vi "Initialize_Filtering_Settings-3.vi"(1 "Sigma #2":dbl, 2 "Sigma #1":dbl) -> (0 "[OUT] Filtering Settings":T1)   [LabVIEW 2013]
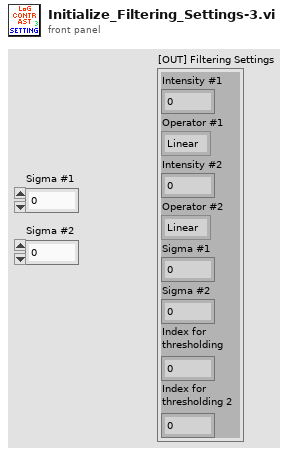
[diagram p1: front panel]
types:
  T1 = cluster{"Intensity #1":sgl, "Operator #1":enum32{"Linear", "Log", "Exp", "Square", "Square root", "Power X", "Power 1/X"}, "Intensity #2":sgl, "Operator #2":enum32{"Linear", "Log", "Exp", "Square", "Square root", "Power X", "Power 1/X"}, "Sigma #1":dbl, "Sigma #2":dbl, "Index for \nthresholding":u8, "Index for \nthresholding 2":u8}
  T2 = enum32{"Linear", "Log", "Exp", "Square", "Square root", "Power X", "Power 1/X"}
  T3 = cluster{"Intensity #1":sgl, "Operator #1":enum32{"Linear", "Log", "Exp", "Square", "Square root", "Power X", "Power 1/X"}, "Intensity #2":sgl, "Operator #2":enum32{"Linear", "Log", "Exp", "Square", "Square root", "Power X", "Power 1/X"}, "Sigma #1":dbl, "Sigma #2":dbl, "Index for \nthresholding":i8, "Index for \nthresholding 2":i8}
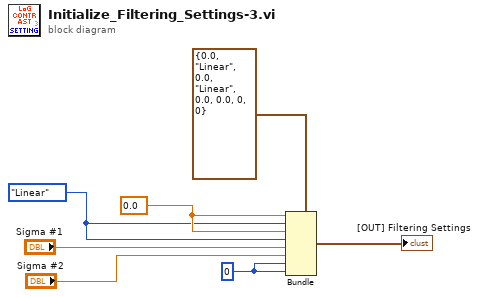
[diagram p0: block diagram]
diagram:
  w2 = i8 0 ("Index for \nthresholding")
  w6 = T2."Linear" ("Operator 3")
  w7 = sgl 0.0 ("Intensity Increase 3")
  n1 = Bundle(cluster=T3 {"Intensity #1"=0.0, "Operator #1"=enum."Linear", "Intensity #2"=0.0, "Operator #2"=enum."Linear", "Sigma #1"=0.0, "Sigma #2"=0.0, "Index for \nthresholding"=0, "Index for \nthresholding 2"=0} ("Image Settings"), "Intensity #1"=w7, "Operator #1"=w6, "Intensity #2"=w7, "Operator #2"=w6, "Sigma #1"="Sigma #1", "Sigma #2"="Sigma #2", "Index for \nthresholding"=w2, "Index for \nthresholding 2"=w2) -> (→"[OUT] Filtering Settings":T3)
